vi "[FPGA] First Order Low Pass Filter Multichannel with Alpha terminal (FLOAT).vi"(0 "x":sgl, 1 "Channel #":u32, 2 "reset":bool, 3 "enable":bool=TRUE, 5 "LPF alpha":sgl=0.0005) -> (4 "filtered x":sgl format="%.2f")   [LabVIEW 2015]
uses:
  <vilib>/rvi/DataTransferAndStorage/Container/Common/niFpgaContainerGetUniqueNameForEmu.vi
  <vilib>/rvi/DataTransferAndStorage/Container/Common/niFpgaContainerSetEmuInfo.vi
  <vilib>/rvi/eio/common/nirviEmuReportErrorAndStop.vi
  <vilib>/rvi/DataTransferAndStorage/Container/Common/niFpgaContainerExecOnDevCompGetState.vi
  <vilib>/rvi/Emulation/niFpgaEmulationIsFPGAContextNoSignature.vi
  <vilib>/rvi/Emulation/niFpgaProcessEmulError.vi
  <vilib>/rvi/Emulation/niFpgaSctlEmulationGetInTimedLoop.vi
  <vilib>/rvi/errors/nirviReportUnexpectedCaseInternalError (U32).vi
  <vilib>/rvi/Memory/Memory_Emulation/niFpgaMemoryEmulationCacheClearOnFirstRun.vi
  <vilib>/rvi/Memory/Memory_Emulation/nirvimemoryEmulationManagerCache_MakeExclusive.vi
  <vilib>/rvi/Memory/Memory_Emulation/niFpgaMemoryEmulationValidateCache.vi
  <vilib>/rvi/Memory/Memory_Emulation/nirvimemoryEmulationManagerCache_InsertValue.vi
  <vilib>/Utility/error.llb/Clear Errors.vi
  <vilib>/rvi/Memory/Memory_Emulation/nirvimemoryEmulationManagerCache_ReleaseExclusive.vi
  <vilib>/rvi/Memory/Memory_Emulation/nirvimemoryEmulationManagerCache_GetValue.vi
  <vilib>/rvi/Memory/Memory_Emulation/nirvimemoryEmulationManagerCache_SetValue.vi
  <vilib>/rvi/Emulation/niFpgaSctlEmulationResourceMgr.vi
  Floating Point/Polymorphic subVIs/Subtract 00.vi
  Floating Point/Polymorphic subVIs/Multiply 00.vi
  Floating Point/Polymorphic subVIs/Add 00.vi
  <vilib>/rvi/LocalResourceManager/LocalResourceManager.xnode
  <vilib>/rvi/DataTransferAndStorage/Container/XNode/niFpgaContainer.xnode
  <vilib>/rvi/Memory/Memory_Emulation/niFpgaMemoryEmulationRefIn.vi
panel:
  # "LPF alpha = dT/(tau+dT) = 1-1/(2*dT*fc*pi+1)"
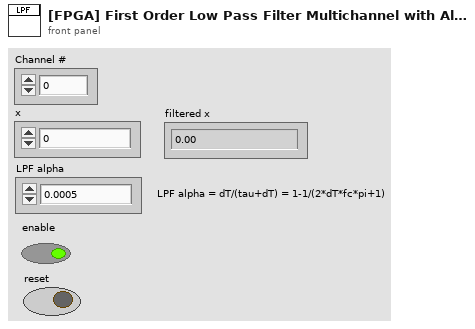
[diagram p1: front panel]
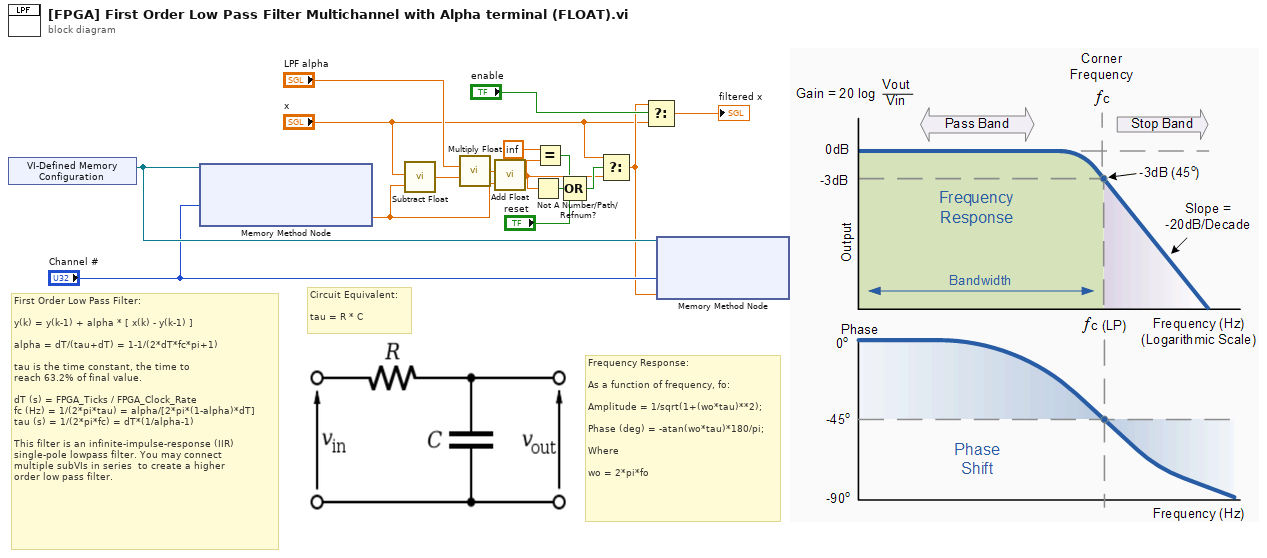
[diagram p0: block diagram]
diagram:
  # "Frequency Response:\n\nAs a function of frequency, fo: \n\nAmplitude = 1/sqrt(1+(wo*tau)**2);\n\nPhase (deg) = -atan(wo*tau)*180/pi;\n\nWhere\n\nwo = 2*pi*fo"
  # "Circuit Equivalent:\n\ntau = R * C"
  # "First Order Low Pass Filter:\n\ny(k) = y(k-1) + alpha * [ x(k) - y(k-1) ]\n\nalpha = dT/(tau+dT) = 1-1/(2*dT*fc*pi+1)\n\ntau is the time constant, the time to \nreach 63.2% of final value.\n\ndT (s) = FPGA_Ticks / FPGA_Clock_Rate\nfc (Hz) = 1/(2*pi*tau) = alpha/[2*pi*(1-alpha)*dT] \ntau (s) = 1/(2*pi*fc) = dT*(1/alpha-1)\n\nThis filter is an infinite-impulse-response (IIR)\nsingle-pole lowpass filter. You may connect \nmultiple subVIs in series  to create a higher \norder low pass filter."
  n1 = xnode ("VI-Defined Memory Configuration")() -> ("Memory Out"=w13:refnum<k21>)
  n2 = xnode ("Memory Method Node")("Address"="Channel #", "Memory In"=w13) -> ("Data"=w12:sgl)  [unwired: 1 out]
  n3 = call-poly "Subtract Float.vi"("y"=w12, "x"="x") -> ("x*y"=w16:sgl)
  n4 = call-poly "Multiply Float.vi"("y"=w16, "x"="LPF alpha") -> ("x*y"=w11:sgl)
  n5 = call-poly "Add Float.vi"("y"=w12, "x"=w11) -> ("x+y"=w5:sgl)
  n6 = Not A Number/Path/Refnum?(number/path/refnum=w5) -> (NaN/Path/Refnum?=w8:bool)
  n7 = Equal?(x=sgl inf, y=w5) -> (x = y?=w3:bool)
  n8 = Compound Arithmetic op=OR(w3, w8, "reset") -> (w6:bool)
  n9 = Select(t="x", s=w6, f=w5) -> (s? t:f=w7:sgl)
  n10 = Select(t=w7, s="enable", f="x") -> (s? t:f=→"filtered x":sgl)
  n11 = xnode ("Memory Method Node")("Address"="Channel #", "Data"=w7, "Memory In"=w13) -> ()  [unwired: 1 out]
